vi "Elevator.vi"() -> ()   [LabVIEW 2013]
panel:
  in  "?":bool
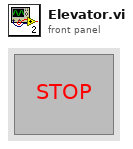
[diagram p1: front panel]
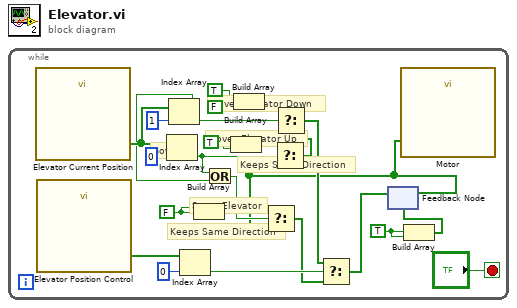
[diagram p0: block diagram]
diagram:
  n1 = while {
    stop <- "?" stop-if-true
    w4 = FALSE
    w10 = TRUE
    w15 = TRUE
    # "Moves Elevator Up"
    # "Keeps Same Direction"
    # "Keeps Same Direction"
    # "Stops Elevator"
    # "Moves Elevator Down"
    # "Bottom"
    # "Top"
    n2 = call "Elevator Current Position"() -> ("data"=w22:bool[])  [unwired: 17 in, 2 out]
    n3 = call "Elevator Position Control"() -> ("data"=w20:bool[])  [unwired: 17 in, 2 out]
    n4 = Index Array(array=w22, index=0) -> (element=w7:bool)
    n5 = Index Array(array=w22, index=1) -> (element=w8:bool)
    n6 = Index Array(array=w20, index=0) -> (element=w19:bool)
    n7 = Build Array(w4, w4) -> (w3:bool[])
    n8 = Or(x=w7, y=w8) -> (x .or. y?=w5:bool)
    n9 = Build Array(w15, w15) -> (w14:bool[])
    n10 = Build Array(TRUE, FALSE) -> (w16:bool[])
    n11 = Build Array(w10, w10) -> (w9:bool[])
    n12 = feedback #1(w9) -> (w1:bool[])
    n13 = Select(t=w3, s=w5, f=w1) -> (s? t:f=w2:bool[])
    n14 = Select(t=w14, s=w7, f=w1) -> (s? t:f=w13:bool[])
    n15 = Select(t=w16, s=w8, f=w13) -> (s? t:f=w12:bool[])
    n16 = Select(t=w12, s=w19, f=w2) -> (s? t:f=w11:bool[])
    n17 = feedback-in #1(w11) -> ()
    n18 = call "Motor"("data"=w1) -> ()  [unwired: 17 in, 2 out]
  }
